vi "TCP_TB_RMW.vi"(0 "REGISTER":string="REGSTR01", 1 "TB IP ADDRESS":string="192.168.0.100", 2 "Bit Bumber":i32, 3 "Connection ID IN":refnum<k5>, 4 "error in (no error)":errorcluster, 5 "Value 1 (TRUE)":bool=TRUE) -> (6 "READ":string, 7 "WRITE":string, 8 "error out":errorcluster)   [LabVIEW 2013]
panel:
  # "INPUTS / CONTROL"
  # "OUTPUTS / RESULT"
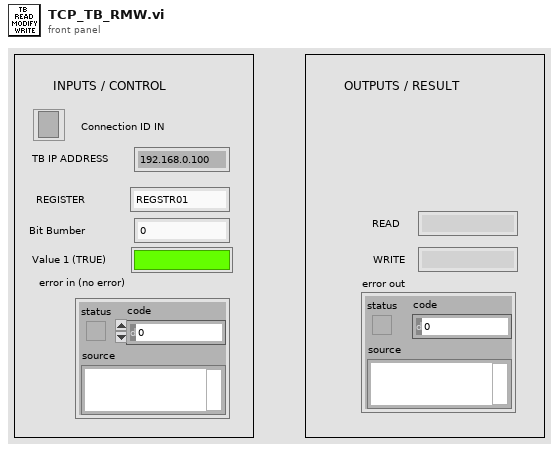
[diagram p1: front panel]
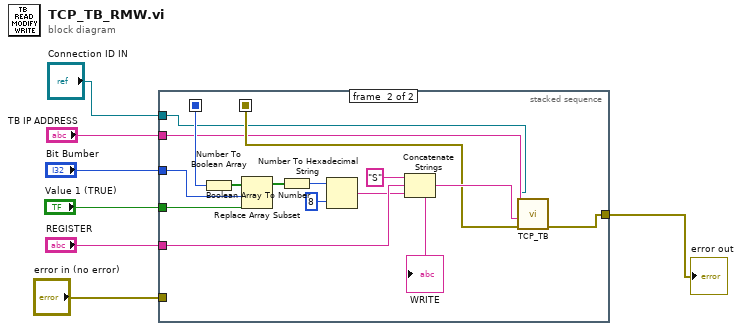
[diagram p0: block diagram]
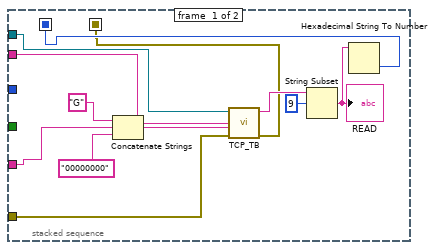
[diagram p2: hidden frame]
diagram:
  n1 = stacked-sequence {
    seq-local: [w10 _] -> [_ w34]
    seq-local: [w9 _] -> [_ w23]
    tunnel: "TB IP ADDRESS" -> [w19 w21]
    tunnel: "error in (no error)" -> [w18 _]
    tunnel: [_ w22] -> w5
    tunnel: "Bit Bumber" -> [_ w32]
    tunnel: "Value 1 (TRUE)" -> [_ w31]
    tunnel: "REGISTER" -> [w15 w26]
    tunnel: "Connection ID IN" -> [w8 w20]
    frame #0 {
      n2 = Concatenate Strings("G" ("COMMAND"), w15, "00000000" ("COMMAND")) -> (w17:string)
      n3 = call "TCP_TB.vi"("IP ADDRESS"=w19, "error in (no error)"=w18, "COMMAND"=w17, "Connection ID IN"=w8) -> ("error out"=w9:errorcluster, "Their Response:"=w12:string)  [unwired: 2 in, 1 out]
      n4 = String Subset(string=w12, offset (0)=9) -> (substring=w11:string)  [unwired: 1 in]
      "READ" <- w11
      n5 = Hexadecimal String To Number(string=w11) -> (number=w10:u32)  [unwired: 2 in, 1 out]
    }
    frame #1 {
      n6 = Number To Boolean Array(number=w34) -> (Boolean array=w33:bool[])
      n7 = Replace Array Subset(array=w33, new element=w31, index=w32) -> (w30:bool[])
      n8 = Boolean Array To Number(Boolean array=w30) -> (number=w29:u32)
      n9 = Number To Hexadecimal String(1:i16 8 ("width (-)"), 2:w29) -> (0:w24:string)
      "WRITE" <- w24
      n10 = Concatenate Strings("S", w26, w24) -> (w25:string)
      n11 = call "TCP_TB.vi"("IP ADDRESS"=w21, "error in (no error)"=w23, "COMMAND"=w25, "Connection ID IN"=w20) -> ("error out"=w22:errorcluster)  [unwired: 2 in, 2 out]
    }
  }
  "error out" <- w5
